vi "Calc Init.vi"(8 "error in (no error)":errorcluster, 10 "Config":refnum<class "Channel Config.lvclass">, 11 "Tare Calc in":refnum<class "Tare Calc.lvclass">) -> (0 "error out":errorcluster, 3 "Tare Calc out":refnum<class "Tare Calc.lvclass">)   [LabVIEW 2020, in "VolatusCalcs.lvlib" / "Tare Calc.lvclass"]
uses:
  Tare Calc.lvclass
  Tare Calc.lvclass/Tare Calc.ctl
  VolatusConfig/VolatusConfigElement/VolatusConfigElement.lvclass
  lv-cdm/CDM-Config/Config Element/Config Element.lvclass
  lv-cdm/CDM-Config/Config Filter/Config Lookup.lvclass
  VolatusConfig/Channel/Channel Config.lvclass
  C:/dev/lv20CE/relink/lv-volatus/VolatusConfig/VolatusConfigElement/VolatusConfigElement.lvclass
  C:/dev/lv20CE/relink/lv-volatus/VolatusConfig/Channel/Channel Config.lvclass
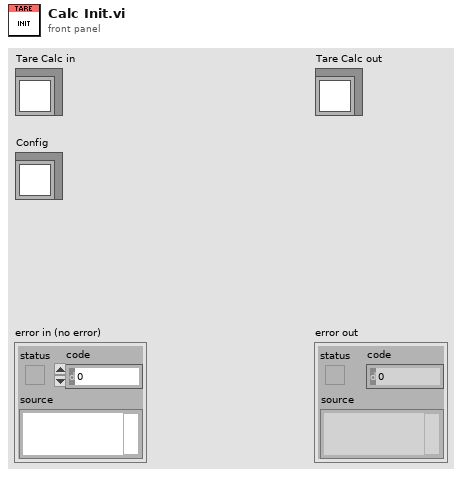
[diagram p1: front panel]
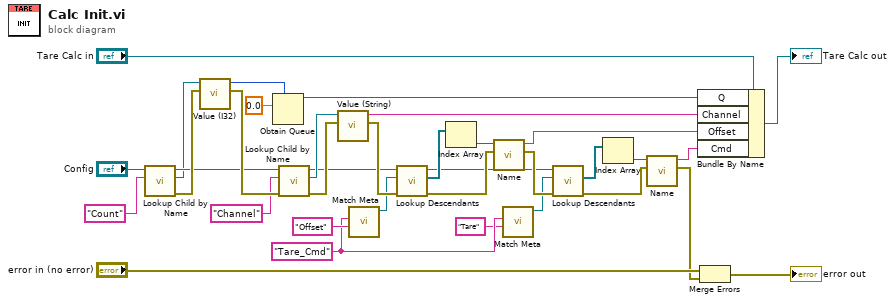
[diagram p0: block diagram]
diagram:
  w20 = "Tare_Cmd" ("Name")
  n1 = call "Lookup Child by Name.vi"("Child Name"="Count", "VolatusConfigElement in"="Config") -> ("error out"=w33:errorcluster, "Child"=w27:refnum<class "Config Element.lvclass">, "VolatusConfigElement out"=w28:refnum<class "Channel Config.lvclass">)  [unwired: 6 in, 1 out]
  n2 = call "Value (I32).vi"("error in (no error)"=w33, "Config Element in"=w27) -> ("error out"=w34:errorcluster, "I32 Value"=w25:i32)  [unwired: 8 in]
  n3 = Obtain Queue(max queue size (-1, unlimited)=w25, element data type=0.0) -> (queue out=w7:refnum<queue>)  [unwired: 3 in, 2 out]
  n4 = call "Lookup Child by Name.vi"("error in (no error)"=w34, "Child Name"="Channel", "VolatusConfigElement in"=w28) -> ("error out"=w22:errorcluster, "Child"=w23:refnum<class "Config Element.lvclass">, "VolatusConfigElement out"=w18:refnum<class "Channel Config.lvclass">)  [unwired: 5 in, 1 out]
  n5 = call "Value (String).vi"("error in (no error)"=w22, "Config Element in"=w23) -> ("error out"=w35:errorcluster, "String Value"=w6:string)  [unwired: 8 in]
  n6 = call "Match Meta.vi"("Value (Any)"="Offset", "Name"=w20) -> ("Config Lookup out"=w17:refnum<class "Config Lookup.lvclass">)  [unwired: 8 in, 1 out]
  n7 = call "Lookup Descendants.vi"("error in (no error)"=w35, "Lookup"=w17, "VolatusConfigElement in"=w18) -> ("error out"=w14:errorcluster, "Descendants"=w16:refnum<class "Config Element.lvclass">[], "VolatusConfigElement out"=w11:refnum<class "Channel Config.lvclass">)  [unwired: 6 in]
  n8 = Index Array(array=w16) -> (element=w15:refnum<class "Config Element.lvclass">)  [unwired: 1 in]
  n9 = call "Name.vi"("error in (no error)"=w14, "Config Element in"=w15) -> ("error out"=w13:errorcluster, "Name"=w5:string)  [unwired: 8 in]
  n10 = call "Match Meta.vi"("Value (Any)"="Tare", "Name"=w20) -> ("Config Lookup out"=w12:refnum<class "Config Lookup.lvclass">)  [unwired: 8 in, 1 out]
  n11 = call "Lookup Descendants.vi"("error in (no error)"=w13, "Lookup"=w12, "VolatusConfigElement in"=w11) -> ("error out"=w3:errorcluster, "Descendants"=w9:refnum<class "Config Element.lvclass">[])  [unwired: 6 in, 1 out]
  n12 = Index Array(array=w9) -> (element=w10:refnum<class "Config Element.lvclass">)  [unwired: 1 in]
  n13 = call "Name.vi"("error in (no error)"=w3, "Config Element in"=w10) -> ("error out"=w1:errorcluster, "Name"=w4:string)  [unwired: 8 in]
  n14 = Bundle By Name(cluster="Tare Calc in", "Q"=w7, "Channel"=w6, "Offset"=w5, "Cmd"=w4) -> (→"Tare Calc out":refnum<class "Tare Calc.lvclass">)
  n15 = Merge Errors("error in (no error)", w1) -> (→"error out":errorcluster)
